vi "Read SettingsFilename.vi"(8 "error in (no error)":errorcluster, 11 "ProgramSettings in":refnum<class "ProgramSettings.lvclass">) -> (0 "error out":errorcluster, 2 "SettingsFilename":string, 3 "ProgramSettings out":refnum<class "ProgramSettings.lvclass">)   [LabVIEW 2019, in "ProgramSettings.lvclass"]
uses:
  ProgramSettings.lvclass
  ProgramSettings.lvclass/ProgramSettings.ctl
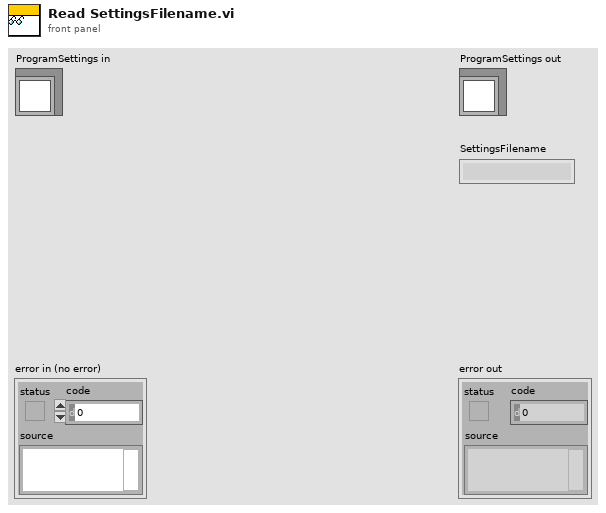
[diagram p1: front panel]
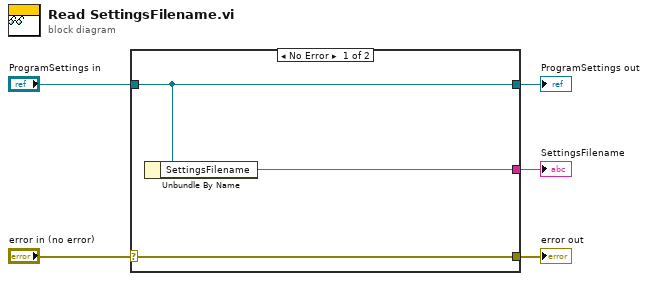
[diagram p0: block diagram]
diagram:
  n1 = case shown="No Error" "error in (no error)" {
    selector: "error in (no error)" -> [w8 w9]
    tunnel: [w8 w9] -> w4
    tunnel: [w7 w10] -> w2
    tunnel: "ProgramSettings in" -> [w7 w10]
    tunnel: [w6 _] -> w1
    frame No Error {
      n2 = Unbundle By Name(w7) -> ("SettingsFilename"=w6:string)
    }
    frame Error {
    }
  }
  "error out" <- w4
  "ProgramSettings out" <- w2
  "SettingsFilename" <- w1
